vi "设定端点.vi"(8 "error in (no error)":errorcluster caption="错误输入（无错误）", 9 "端点B":T1 caption="点", 10 "端点A":T1 caption="点", 11 "直线 输入":refnum<class "直线.lvclass"> caption="DNL_LabVIEW Object in") -> (0 "error out":errorcluster caption="错误输出", 3 "直线 输出":refnum<class "直线.lvclass"> caption="DNL_LabVIEW Object out")   [LabVIEW 2011, in "直线.lvclass"]
uses:
  <vilib>/Utility/miscctls.llb/LVPointDoubleTypeDef.ctl
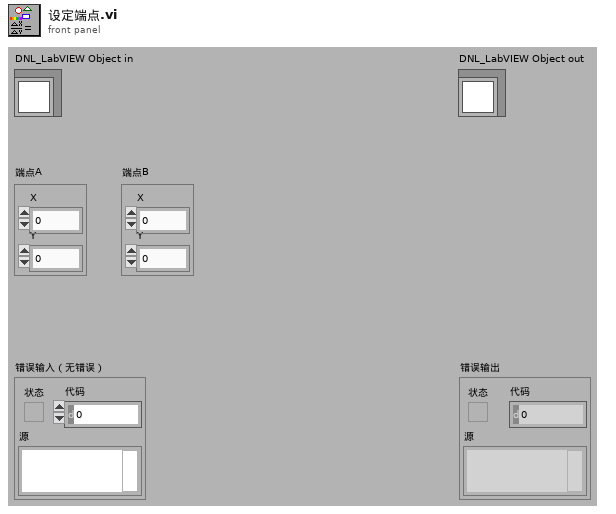
[diagram p1: front panel]
types:
  T1 = typedef "LVPointDoubleTypeDef.ctl" = cluster{"X":dbl, "Y":dbl}
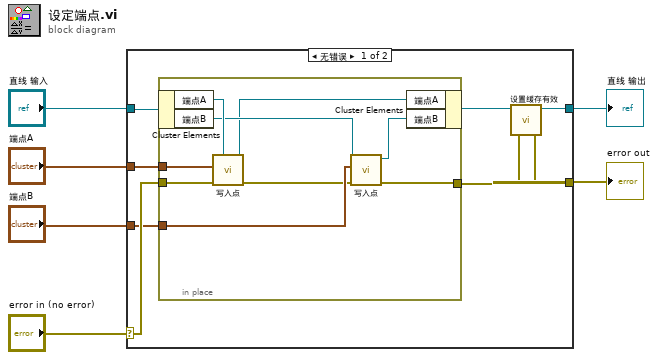
[diagram p0: block diagram]
diagram:
  n1 = case shown="无错误" "error in (no error)" {
    selector: "error in (no error)" -> [w12 w25]
    tunnel: [w7 w25] -> w5
    tunnel: [w9 w24] -> w3
    tunnel: "直线 输入" -> [w14 w24]
    tunnel: "端点A" -> [w13 _]
    tunnel: "端点B" -> [w11 _]
    frame No Error {
      n2 = in-place {
        in-place-border: w13 -> [w22]
        in-place-border: w12 -> [w21]
        in-place-border: w11 -> [w19]
        in-place-border: [w17] -> w8
        n3 = in-place-cluster #1(w14) -> ("端点A"=w23:refnum<class "点.lvclass">, "端点B"=w20:refnum<class "点.lvclass">)
        n4 = call "写入点.vi"("error in (no error)"=w21, "点"=w22, "点输入"=w23) -> ("error out"=w16:errorcluster, "点输出"=w15:refnum<class "点.lvclass">)  [unwired: 7 in]
        n5 = call "写入点.vi"("error in (no error)"=w16, "点"=w19, "点输入"=w20) -> ("error out"=w17:errorcluster, "点输出"=w18:refnum<class "点.lvclass">)  [unwired: 7 in]
        n6 = in-place-cluster #1("端点A"=w15, "端点B"=w18) -> (w10:refnum<class "直线.lvclass">)
      }
      n7 = call "设置缓存有效.vi"("error in (no error)"=w8, "图形 输入"=w10) -> ("error out"=w7:errorcluster, "图形 输出"=w9:refnum<class "直线.lvclass">)  [unwired: 8 in]
    }
    frame Error {
    }
  }
  "error out" <- w5
  "直线 输出" <- w3
